vi "Schier lab scheduler 2.vi"(10 "Load Experimental Parameters":path, 11 "External Stop":refnum<vi>) -> (3 "doQueue2":refnum<queue>)   [LabVIEW 2013]
panel:
  out "Event Data":dbl[][](array[numeric])
  out "Event times":string[](array[string])
  out "current time":string
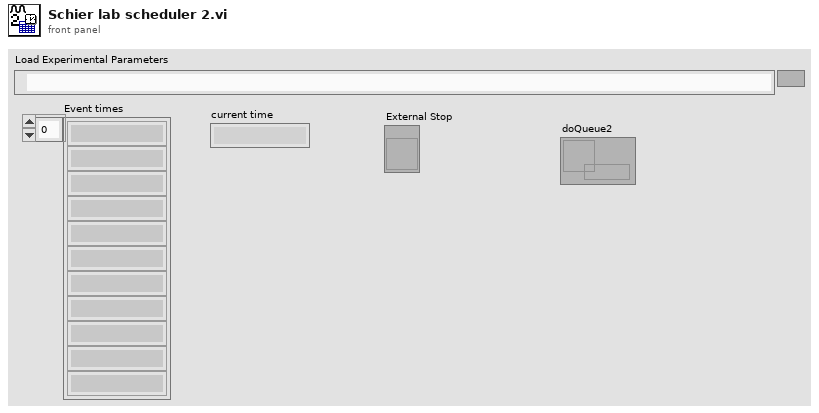
[diagram p1: front panel]
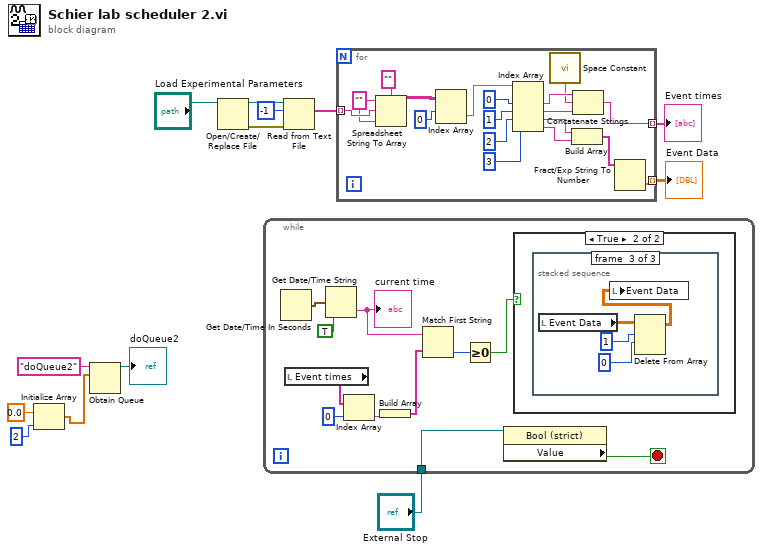
[diagram p0: block diagram]
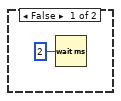
[diagram p2: hidden frame]
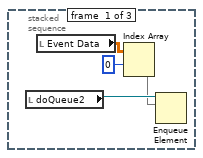
[diagram p3: hidden frame]
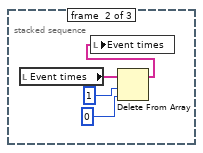
[diagram p4: hidden frame]
diagram:
  n1 = Initialize Array(0.0 ("element"), 2 ("dimension size")) -> (w3:dbl[])
  n2 = Obtain Queue(name (unnamed)="doQueue2", element data type=w3) -> (queue out=→"doQueue2":refnum<queue>)  [unwired: 3 in, 2 out]
  n3 = Open/Create/Replace File(file path (use dialog)="Load Experimental Parameters") -> (refnum out=w12:refnum<file>, error out=w11:errorcluster)  [unwired: 5 in, 1 out]
  n4 = while {
    tunnel: "External Stop" -> [w18]
    stop <- w19 stop-if-true
    n5 = Get Date/Time In Seconds() -> (seconds since 1Jan1904=w24:timestamp)
    n6 = local read "Event times"() -> (w15:string[])
    n7 = Get Date/Time String(seconds (now)=w24, want seconds? (F)=TRUE) -> (time string=w22:string)  [unwired: 1 in, 1 out]
    "current time" <- w22
    n8 = Index Array(array=w15, index=0) -> (element=w16:string)
    n9 = Build Array(w16) -> (w14:string[])
    n10 = Match First String(2:w14, 3:w22) -> (0:w20:i32)  [unwired: 1 out]
    n11 = Greater Or Equal To 0?(x=w20) -> (x >= 0?=w21:bool)
    n12 = property class="Bool (strict)"(reference=w18) -> ("Value"=w19:bool)  [unwired: 1 in, 2 out]
    n13 = case shown="True" w21 {
      frame False {
        n14 = Wait (ms)(milliseconds to wait=u32 2) -> ()  [unwired: 1 out]
      }
      frame True {
        n15 = stacked-sequence {
          frame #0 {
            n16 = local read "doQueue2"() -> (w28:refnum<queue>)
            n17 = local read "Event Data"() -> (w29:dbl[][])
            n18 = Index Array(array=w29, index (row)=0) -> (element=w27:dbl[])  [unwired: 1 in]
            n19 = Enqueue Element(queue=w28, element=w27) -> ()  [unwired: 2 in, 3 out]
          }
          frame #1 {
            n20 = local read "Event times"() -> (w31:string[])
            n21 = Delete From Array(array=w31, length=1, index=0) -> (array with subset deleted=w33:string[])  [unwired: 1 out]
            n22 = local write "Event times"(w33) -> ()
          }
          frame #2 {
            n23 = local read "Event Data"() -> (w36:dbl[][])
            n24 = Delete From Array(array=w36, length=1, index (row)=0 ("index")) -> (array with subset deleted=w34:dbl[][])  [unwired: 1 in, 1 out]
            n25 = local write "Event Data"(w34) -> ()
          }
        }
      }
    }
  }
  n26 = Read from Text File(file (use dialog)=w12, count=-1, error in=w11) -> (text=w9:string[])  [unwired: 1 in, 3 out]
  n27 = for {
    tunnel: w9 -> [w54] mode=indexing
    tunnel: [w42] -> w8 mode=indexing
    tunnel: [w38] -> w7 mode=indexing
    w53 = "" ("format string")
    n28 = Spreadsheet String To Array(delimiter (Tab)="", format string=w53, spreadsheet string=w54, array type (2D Dbl)=w53) -> (array=w52:string[][])
    n29 = Index Array(array=w52, index (row)=0 ("disabled index (col)")) -> (element=w50:string[])  [unwired: 1 in]
    n30 = Index Array(array=w50, index #1=0 ("index"), index #2=1 ("index"), index #3=2 ("index"), index #4=3 ("index")) -> (element #1=w45:string, element #2=w44:string, element #3=w41:string, element #4=w40:string)
    n31 = call <vilib>:"Space Constant.vi"() -> ("String"=w43:string)
    n32 = Build Array(w41, w40) -> (w39:string[])
    n33 = Concatenate Strings(w45, w43, w44) -> (w42:string)
    n34 = Fract/Exp String To Number(string=w39) -> (number=w38:dbl[])  [unwired: 3 in, 1 out]
  }
  "Event times" <- w8
  "Event Data" <- w7
